vi "to string.vi"(8 "error in":errorcluster, 11 "tag bus configurable plugin module configuration in":refnum<class "tag bus configurable plugin module configuration.lvclass">) -> (0 "error out":errorcluster, 1 "data":string, 2 "version":string, 3 "tag bus configurable plugin module configuration out":refnum<class "tag bus configurable plugin module configuration.lvclass">)   [LabVIEW 2013, in "tag bus configurable plugin module configuration.lvclass"]
doc: "Provides an interface for saving a module configuration to a file or other serialized data source. It is recommended that all children of this class store data in two sets--data required for its own initialization, and any data required for parent initialization--and that each implementation uses the <b>Call Parent Method</b> primitive to serialize parent information."
uses:
  tag bus configurable plugin module configuration.lvclass
  current version.vi
  <vilib>/NI/Tag Bus Module Framework/module configuration/TBM module configuration.lvclass
  <vilib>/NI/Tag Bus Module Framework/channel/TBM channel.lvclass
  <vilib>/NI/Configuration Framework/serializable configuration/NISE_CEF_serializable configuration.lvclass
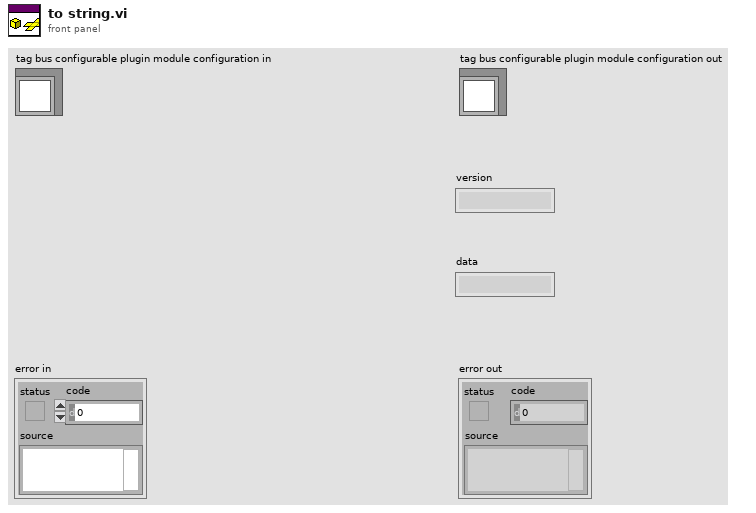
[diagram p1: front panel]
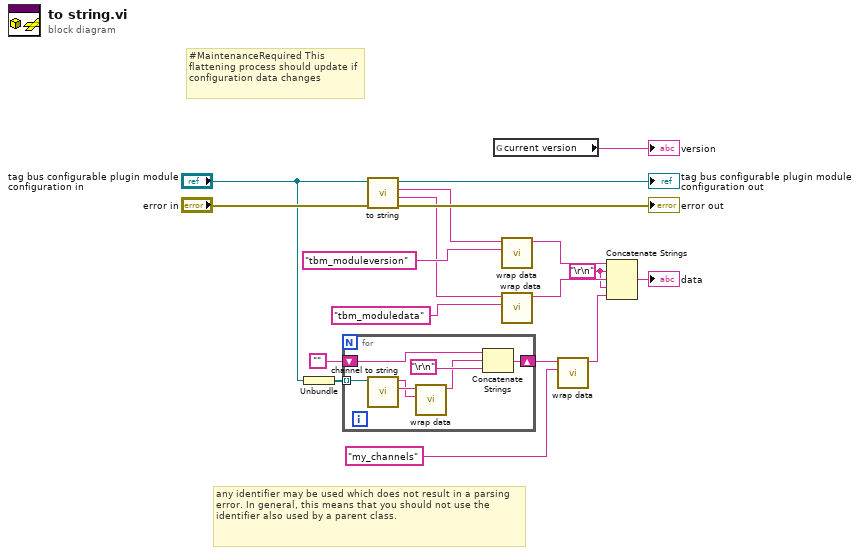
[diagram p0: block diagram]
diagram:
  w1 = "\r\n"
  # "any identifier may be used which does not result in a parsing error. In general, this means that you should not use the identifier also used by a parent class."
  # "#MaintenanceRequired This flattening process should update if configuration data changes"
  n1 = Unbundle("tag bus configurable plugin module configuration in") -> (w4:refnum<class "TBM channel.lvclass">[])
  n2 = for {
    tunnel: w4 -> [w25] mode=indexing
    shift-right: [w21] -> w2
    shift-left: "" -> [w20]
    n3 = call <vilib>:"channel to string.vi"("channel in"=w25) -> ("channel data"=w24:string, "identifier"=w23:string)  [unwired: 9 in]
    n4 = call <vilib>:"wrap data.vi"("identifier"=w23, "data to wrap"=w24) -> ("wrapped data"=w19:string)  [unwired: 9 in]
    n5 = Concatenate Strings(w20, w19, "\r\n") -> (w21:string)
  }
  n6 = call-parent "to string.vi"("error in"="error in", "module configuration in"="tag bus configurable plugin module configuration in") -> ("error out"=→"error out":errorcluster, "data"=w9:string, "version"=w10:string, "module configuration out"=→"tag bus configurable plugin module configuration out":refnum<class "tag bus configurable plugin module configuration.lvclass">)  [unwired: 6 in]
  n7 = global read "current version.vi" "current version"() -> (→"version":string)
  n8 = call <vilib>:"wrap data.vi"("identifier"="tbm_moduleversion" ("additional identifier"), "data to wrap"=w10) -> ("wrapped data"=w12:string)  [unwired: 9 in]
  n9 = call <vilib>:"wrap data.vi"("identifier"="tbm_moduledata" ("additional identifier"), "data to wrap"=w9) -> ("wrapped data"=w11:string)  [unwired: 9 in]
  n10 = call <vilib>:"wrap data.vi"("identifier"="my_channels" ("additional identifier"), "data to wrap"=w2) -> ("wrapped data"=w6:string)  [unwired: 9 in]
  n11 = Concatenate Strings(w12, w1, w11, w1, w6) -> (→"data":string)
